vi "SimDuck.vi"() -> ()   [LabVIEW 2013]
uses:
  MallardDuck/MallardDuck.lvclass
  RedhearDuck/RedheadDuck.lvclass
  RubberDuck/RubberDuck.lvclass
  ModelDuck/ModelDuck.lvclass
  Duck/Duck.lvclass
panel:
  out "鴨子的描述(依介面)":string
  in  "什麼鴨?":enum16{"綠頭鴨", "紅頭鴨", "橡皮鴨", "模型鴨"}(ring)
  out "鴨子的描述(依繼承)":string
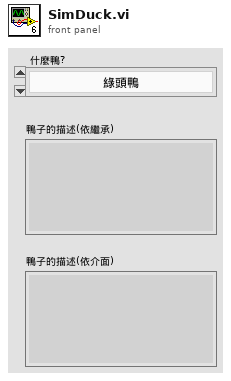
[diagram p1: front panel]
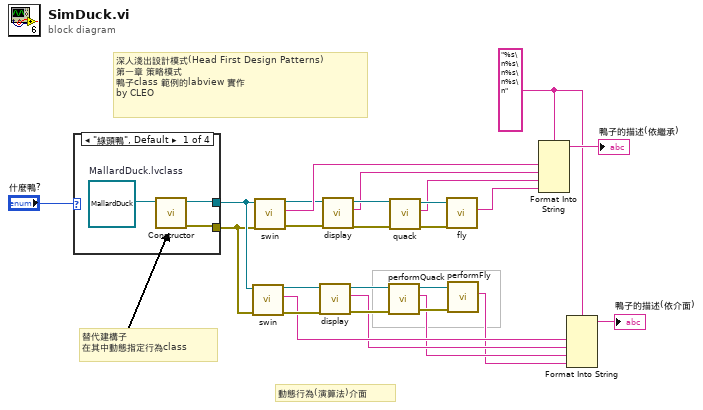
[diagram p0: block diagram]
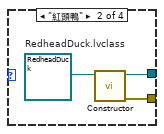
[diagram p2: hidden frame]
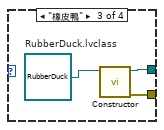
[diagram p3: hidden frame]
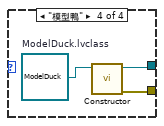
[diagram p4: hidden frame]
diagram:
  w1 = "%s\n%s\n%s\n%s\n" ("format string")
  # "深人淺出設計模式(Head First Design Patterns)\n第一章 策略模式\n鴨子class 範例的labview 實作\nby CLEO"
  # "替代建構子\n在其中動態指定行為class"
  # "動態行為(演算法)介面"
  n1 = case shown="\"綠頭鴨\", Default" "什麼鴨?" {
    tunnel: [w29 w32 w34 w37] -> w22
    tunnel: [w28 w30 w33 w36] -> w21
    frame "綠頭鴨", Default {
      w27 = refnum<class "MallardDuck.lvclass"> refnum  # MallardDuck.lvclass
      n2 = call-dynamic "Constructor.vi"("MallardDuck in"=w27) -> ("error out"=w28:errorcluster, "MallardDuck out"=w29:refnum<class "MallardDuck.lvclass">)  [unwired: 9 in]
    }
    frame "紅頭鴨" {
      w31 = refnum<class "RedheadDuck.lvclass"> refnum  # RedheadDuck.lvclass
      n3 = call-dynamic "Constructor.vi"("RedheadDuck in"=w31) -> ("error out"=w30:errorcluster, "RedheadDuck out"=w32:refnum<class "RedheadDuck.lvclass">)  [unwired: 9 in]
    }
    frame "橡皮鴨" {
      w35 = refnum<class "RubberDuck.lvclass"> refnum  # RubberDuck.lvclass
      n4 = call-dynamic "Constructor.vi"("RubberDuck in"=w35) -> ("error out"=w33:errorcluster, "RubberDuck out"=w34:refnum<class "RubberDuck.lvclass">)  [unwired: 9 in]
    }
    frame "模型鴨" {
      w38 = refnum<class "ModelDuck.lvclass"> refnum  # ModelDuck.lvclass
      n5 = call-dynamic "Constructor.vi"("ModelDuck in"=w38) -> ("error out"=w36:errorcluster, "ModelDuck out"=w37:refnum<class "ModelDuck.lvclass">)  [unwired: 9 in]
    }
  }
  n6 = call-dynamic "swin.vi"("error in (no error)"=w21, "Duck in"=w22) -> ("error out"=w11:errorcluster, "State"=w5:string, "Duck out"=w12:refnum<class "Duck.lvclass">)  [unwired: 7 in]
  n7 = call-dynamic "swin.vi"("error in (no error)"=w21, "Duck in"=w22) -> ("error out"=w19:errorcluster, "State"=w26:string, "Duck out"=w20:refnum<class "Duck.lvclass">)  [unwired: 7 in]
  n8 = call-dynamic "display.vi"("error in (no error)"=w11, "Duck in"=w12) -> ("error out"=w7:errorcluster, "State"=w4:string, "Duck out"=w10:refnum<class "Duck.lvclass">)  [unwired: 7 in]
  n9 = call-dynamic "display.vi"("error in (no error)"=w19, "Duck in"=w20) -> ("error out"=w17:errorcluster, "State"=w16:string, "Duck out"=w18:refnum<class "Duck.lvclass">)  [unwired: 7 in]
  n10 = call-dynamic "performQuack.vi"("error in (no error)"=w7, "Duck in"=w10) -> ("error out"=w8:errorcluster, "State"=w3:string, "Duck out"=w9:refnum<class "Duck.lvclass">)  [unwired: 7 in]
  n11 = call-dynamic "quack.vi"("error in (no error)"=w17, "Duck in"=w18) -> ("error out"=w14:errorcluster, "State"=w13:string, "Duck out"=w15:refnum<class "Duck.lvclass">)  [unwired: 7 in]
  n12 = call-dynamic "fly.vi"("error in (no error)"=w14, "Duck in"=w15) -> ("String"=w23:string)  [unwired: 7 in, 2 out]
  n13 = call-dynamic "performFly.vi"("error in (no error)"=w8, "Duck in"=w9) -> ("State"=w2:string)  [unwired: 7 in, 2 out]
  n14 = Format Into String(format string=w1, w26, w16, w13, w23) -> (resulting string=→"鴨子的描述(依繼承)":string)  [unwired: 2 in, 1 out]
  n15 = Format Into String(format string=w1, w5, w4, w3, w2) -> (resulting string=→"鴨子的描述(依介面)":string)  [unwired: 2 in, 1 out]
